vi "Memory.Pointer.Copy.Unsafe.vi"(8 "error in (no error)":errorcluster, 9 "bytes to copy":u64 format="%08x bytes", 10 "dst pointer in":refnum<class "Memory.Pointer.lvclass">, 11 "src pointer in":refnum<class "Memory.Pointer.lvclass">) -> (0 "error out":errorcluster, 1 "bytes to copy":u64 format="%08x bytes", 2 "dst pointer out":refnum<class "Memory.Pointer.lvclass">, 3 "src pointer out":refnum<class "Memory.Pointer.lvclass">)   [LabVIEW 2016, in "Memory.lvlib" / "Memory.Pointer.lvclass"]
doc: "Copies <b>bytes to copy</b> of data from the memory address specified by <b>src pointer</b> to the memory address specified by <b>dst pointer</b>.\n\n<b>Note:</b> This VI is <b>unsafe</b>.\n\nUnsafe means that this function does not have a check to ensure that the size of the requested source memory transfer is inbounds of allocated memory for the destination before peforming a memory read/write. Reading/writing more data to a pointer than it has allocated can corrupt or crash LabVIEW. Only use this VI in scenarios where the <b>dst pointer</b> has been validated to be allocated to a correct size before calling this VI."
uses:
  Memory.Pointer.lvclass
  Memory.Pointer.lvclass/Memory.Pointer.ctl
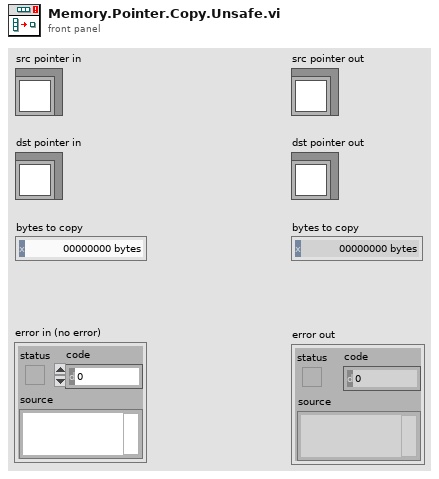
[diagram p1: front panel]
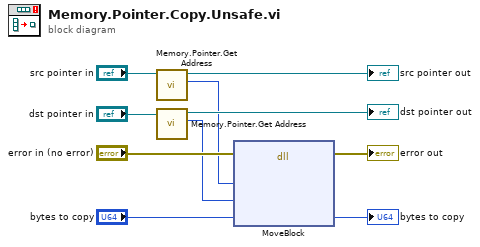
[diagram p0: block diagram]
diagram:
  n1 = call "Memory.Pointer.Get Address.vi"("Pointer in"="src pointer in") -> ("address"=w3:u64, "Pointer out"=→"src pointer out":refnum<class "Memory.Pointer.lvclass">)  [unwired: 8 in, 1 out]
  n2 = call "Memory.Pointer.Get Address.vi"("Pointer in"="dst pointer in") -> ("address"=w4:u64, "Pointer out"=→"dst pointer out":refnum<class "Memory.Pointer.lvclass">)  [unwired: 8 in, 1 out]
  n3 = dll-call lib="LabVIEW" fn="MoveBlock"(error in="error in (no error)", "src"=w3, "dst"=w4, "size"="bytes to copy") -> (error out=→"error out":errorcluster, "size"=→"bytes to copy":u64)  [unwired: 5 in, 1 out]
